vi "iHeartConnector.vi"() -> ()   [LabVIEW 2018]
panel:
  out "Pulse":u16
  out "Sp02":u16
  out "Ticks":u32
  out "Millis":u16
  out "Second":u8
  out "Minute":u8
  out "Hour":u8
  out "Day":u8
  out "Month":u8
  out "Year":u8
  out "Id":string
  out "IR":i32(graph)
  in  "stop":bool
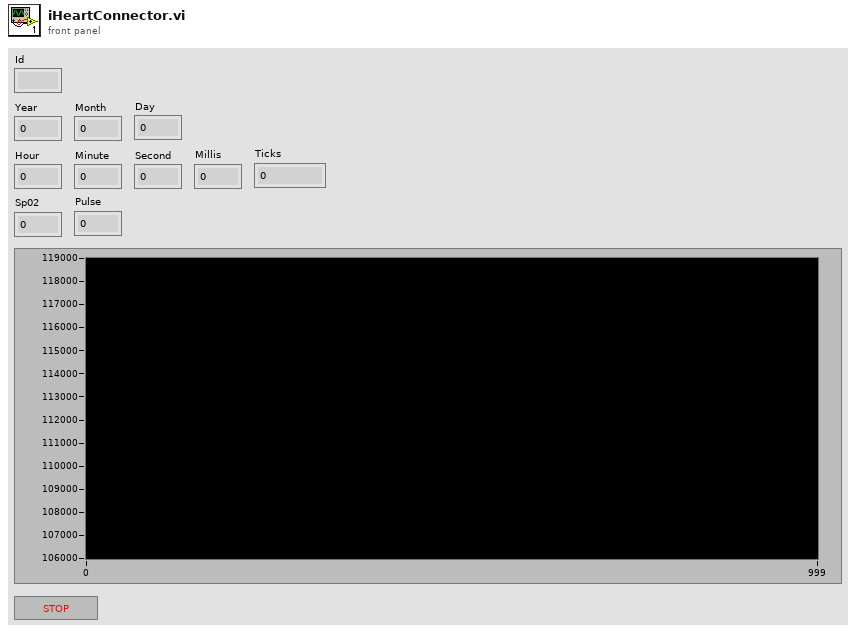
[diagram p1: front panel]
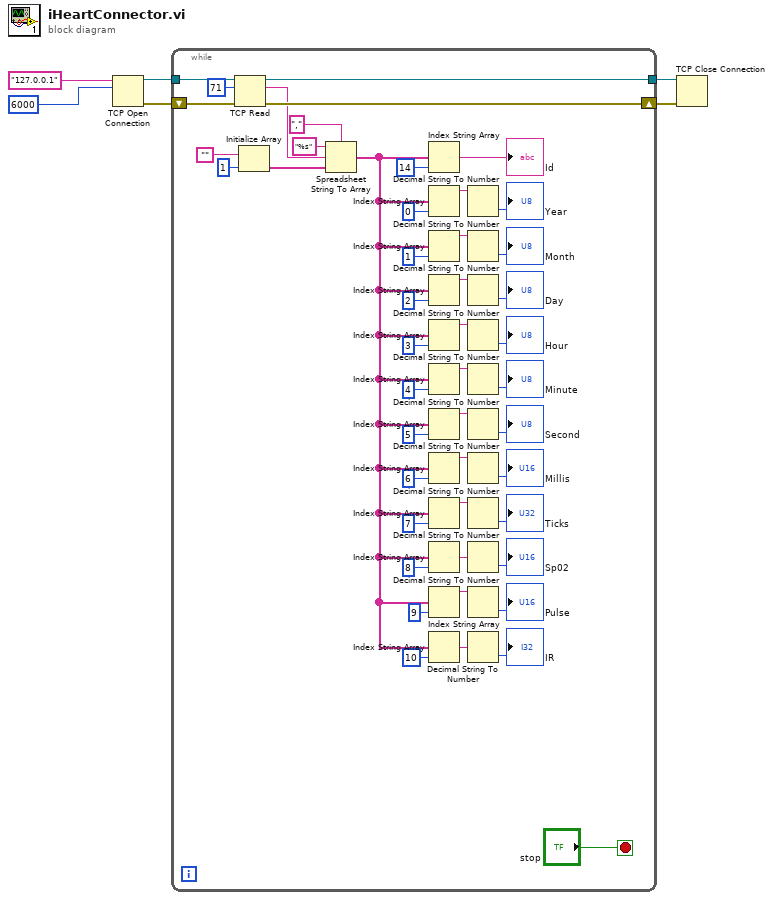
[diagram p0: block diagram]
diagram:
  n1 = TCP Open Connection(address="127.0.0.1", remote port or service name=u16 6000) -> (connection ID=w2:refnum<k5>, error out=w6:errorcluster)  [unwired: 3 in]
  n2 = while {
    shift-right: [w53] -> w5
    shift-left: w6 -> [w54]
    tunnel: w2 -> [w51]
    tunnel: [w50] -> w1
    stop <- "stop" stop-if-true
    n3 = TCP Read(connection ID=w51, bytes to read=71, error in (no error)=w54) -> (connection ID out=w50:refnum<k5>, data out=w48:string, error out=w53:errorcluster)  [unwired: 2 in]
    n4 = Initialize Array("", 1 ("dimension size")) -> (w44:string[])
    n5 = Spreadsheet String To Array(delimiter (Tab)=",", format string="%s", spreadsheet string=w48, array type (2D Dbl)=w44) -> (array=w7:string[])
    n6 = Index String Array(1:14 ("index"), 2:w7) -> (0:→"Id":string)  [unwired: 1 in]
    n7 = Index String Array(1:0 ("index"), 2:w7) -> (0:w36:string)  [unwired: 1 in]
    n8 = Index String Array(1:1 ("index"), 2:w7) -> (0:w33:string)  [unwired: 1 in]
    n9 = Index String Array(1:2 ("index"), 2:w7) -> (0:w30:string)  [unwired: 1 in]
    n10 = Index String Array(1:3 ("index"), 2:w7) -> (0:w27:string)  [unwired: 1 in]
    n11 = Index String Array(1:4 ("index"), 2:w7) -> (0:w24:string)  [unwired: 1 in]
    n12 = Index String Array(1:5 ("index"), 2:w7) -> (0:w21:string)  [unwired: 1 in]
    n13 = Index String Array(1:6 ("index"), 2:w7) -> (0:w17:string)  [unwired: 1 in]
    n14 = Index String Array(1:7 ("index"), 2:w7) -> (0:w14:string)  [unwired: 1 in]
    n15 = Index String Array(1:8 ("index"), 2:w7) -> (0:w11:string)  [unwired: 1 in]
    n16 = Index String Array(1:9 ("index"), 2:w7) -> (0:w8:string)  [unwired: 1 in]
    n17 = Index String Array(1:10 ("index"), 2:w7) -> (0:w38:string)  [unwired: 1 in]
    n18 = Decimal String To Number(string=w36) -> (number=→"Year":i32)  [unwired: 2 in, 1 out]
    n19 = Decimal String To Number(string=w33) -> (number=→"Month":i32)  [unwired: 2 in, 1 out]
    n20 = Decimal String To Number(string=w30) -> (number=→"Day":i32)  [unwired: 2 in, 1 out]
    n21 = Decimal String To Number(string=w27) -> (number=→"Hour":i32)  [unwired: 2 in, 1 out]
    n22 = Decimal String To Number(string=w24) -> (number=→"Minute":i32)  [unwired: 2 in, 1 out]
    n23 = Decimal String To Number(string=w21) -> (number=→"Second":i32)  [unwired: 2 in, 1 out]
    n24 = Decimal String To Number(string=w17) -> (number=→"Millis":i32)  [unwired: 2 in, 1 out]
    n25 = Decimal String To Number(string=w14) -> (number=→"Ticks":i32)  [unwired: 2 in, 1 out]
    n26 = Decimal String To Number(string=w11) -> (number=→"Sp02":i32)  [unwired: 2 in, 1 out]
    n27 = Decimal String To Number(string=w8) -> (number=→"Pulse":i32)  [unwired: 2 in, 1 out]
    n28 = Decimal String To Number(string=w38) -> (number=→"IR":i32)  [unwired: 2 in, 1 out]
  }
  n29 = TCP Close Connection(connection ID=w1, error in (no error)=w5) -> ()  [unwired: 1 in, 2 out]
